vi "bottom stacking.vi"() -> (10 "Done":bool)   [LabVIEW 2014]
uses:
  Bottom Stacking.ctl
  <vilib>/Rock Robotics/WPI/RobotDrive/WPI_RobotDriveGetSetRefNum.vi
panel:
  out "Timer":dbl
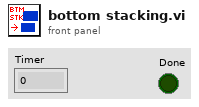
[diagram p1: front panel]
types:
  T1 = typedef "Bottom Stacking.ctl" = enum16{"Tote Raising", "Ejecting", "Un-Ejecting", "Tote Lowering", "Tote Release", "Backing Up"}
  T2 = typedef "WPI_RobotDriveDevRef.ctl" = cluster{"DevStatus":errorcluster, "Motors[]":T3[], "Square Inputs":bool, "Max Output":dbl}
  T3 = typedef "WPI_MotorControlDeviceRef.ctl" = cluster{"DeviceStatus":errorcluster, "Type":T4, "PWM":cluster{"Controller":T5, "PWM Channel":T6, "DeadBand":T7}, "CAN":cluster{"Device Number":u8, "Control Mode":T8, "Semaphore":T9, "Max Vout":dbl, "TalonSRX Control Mode":T10}, "Invert":bool, "TransformRef":T11, "InvTransformRef":T11}
  T4 = typedef "WPI_MotorControlType.ctl" = enum16{"PWM", "CAN", "CANTalonSRX"}
  T5 = typedef "FPGA_TypedefDigitalModule.ctl" = enum16{"Controller 1"}
  T6 = typedef "FPGA_DIOPWMChannel.ctl" = enum8{"PWM 0", "PWM 1", "PWM 2", "PWM 3", "PWM 4", "PWM 5", "PWM 6", "PWM 7", "PWM 8", "PWM 9", "PWM MXP 0", "PWM MXP 1", "PWM MXP 2", "PWM MXP 3", "PWM MXP 4", "PWM MXP 5", "PWM MXP 6", "PWM MXP 7", "PWM MXP 8", "PWM MXP 9", "Invalid"}
  T7 = typedef "WPI_PWMDeadband.ctl" = cluster{"Name":string, "maxPositivePwm":i32, "minPositivePwm":i32, "centerPwm":i32, "maxNegativePwm":i32, "minNegativePwm":i32, "angularRange":u16}
  T8 = typedef "WPI_CANJaguar_ControlMode.ctl" = enum8{"Percent VBus", "Current", "Speed", "Position", "Voltage"}
  T9 = typedef "Semaphore RefNum" = refnum<k1>
  T10 = typedef "WPI_CANTalonSRX_APIControlMode.ctl" = enum8{"Percent VBus", "Speed", "Position", "Slave", "Unchanged / Invalid"}
  T11 = typedef "WPI_PWMTransform_ConPane.ctl" = refnum<vi>
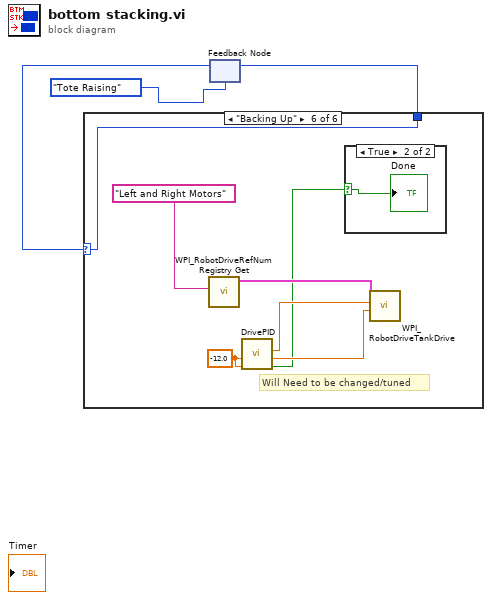
[diagram p0: block diagram]
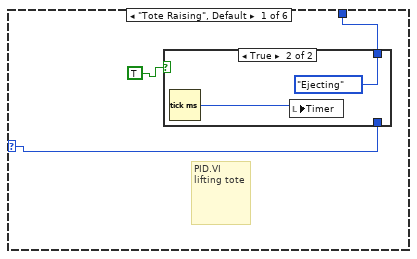
[diagram p2: hidden frame]
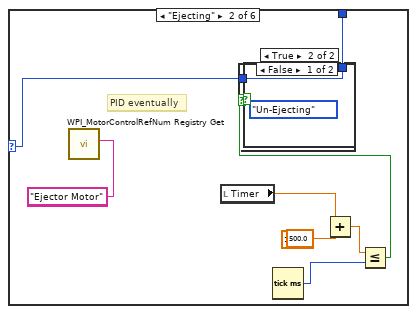
[diagram p4: hidden frame]
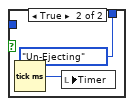
[diagram p5: hidden frame]
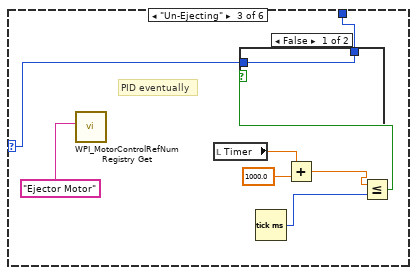
[diagram p7: hidden frame]
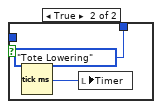
[diagram p8: hidden frame]
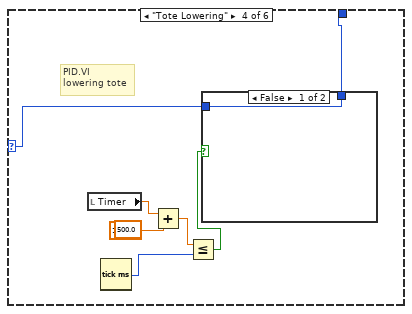
[diagram p9: hidden frame]
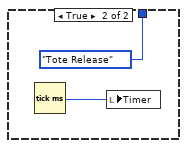
[diagram p10: hidden frame]
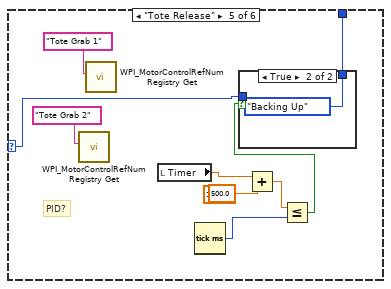
[diagram p11: hidden frame]
diagram:
  n1 = feedback #1(Bottom_Stacking."Tote Raising" ("Bottom Stacking")) -> (w2:T1)
  n2 = case shown="\"Backing Up\"" w2 {
    selector: w2 -> [w5 w10 w27 w37 w49 w58]
    tunnel: [w6 w11 w29 w43 w53 w58] -> w1
    frame "Tote Raising", Default {
      # "PID.VI\nlifting tote"
      n3 = case shown="True" TRUE {
        tunnel: [w7 Bottom_Stacking."Ejecting" ("Bottom Stacking")] -> w6
        tunnel: w5 -> [w7 _]
        frame False {
        }
        frame True {
          n4 = Tick Count (ms)() -> (millisecond timer value=w8:u32)
          n5 = local write "Timer"(w8) -> ()
        }
      }
    }
    frame "Ejecting" {
      (unwired) "Ejector Motor" ("refnum name")
      # "PID eventually"
      # "PID eventually"
      n6 = call <vilib>:"WPI_MotorControlRefNum Registry Get.vi"("refnum name"="Ejector Motor") -> ()  [unwired: 9 in, 2 out]
      n7 = local read "Timer"() -> (w21:dbl)
      n8 = local read "Timer"() -> (w12:dbl)
      n9 = Tick Count (ms)() -> (millisecond timer value=w18:u32)
      n10 = Tick Count (ms)() -> (millisecond timer value=w15:u32)
      n11 = Add(x=w21, y=500.0) -> (x+y=w19:dbl)
      n12 = Add(x=w12, y=1000.0) -> (x+y=w14:dbl)
      n13 = Less Or Equal?(x=w19, y=w18) -> (x <= y?=w17:bool)
      n14 = case shown="True" w17 {
        frame False {
        }
        frame True {
          (unwired) Bottom_Stacking."Un-Ejecting" ("Bottom Stacking")
        }
      }
      n15 = Less Or Equal?(x=w14, y=w15) -> (x <= y?=w16:bool)
      n16 = case shown="False" w16 {
        tunnel: [w23 Bottom_Stacking."Un-Ejecting" ("Bottom Stacking")] -> w11
        tunnel: w10 -> [w23 _]
        frame False {
        }
        frame True {
          n17 = Tick Count (ms)() -> (millisecond timer value=w25:u32)
          n18 = local write "Timer"(w25) -> ()
        }
      }
    }
    frame "Un-Ejecting" {
      # "PID eventually"
      n19 = call <vilib>:"WPI_MotorControlRefNum Registry Get.vi"("refnum name"="Ejector Motor") -> ()  [unwired: 9 in, 2 out]
      n20 = local read "Timer"() -> (w33:dbl)
      n21 = Tick Count (ms)() -> (millisecond timer value=w30:u32)
      n22 = Add(x=w33, y=1000.0) -> (x+y=w31:dbl)
      n23 = Less Or Equal?(x=w31, y=w30) -> (x <= y?=w28:bool)
      n24 = case shown="False" w28 {
        tunnel: [w34 Bottom_Stacking."Tote Lowering" ("Bottom Stacking")] -> w29
        tunnel: w27 -> [w34 _]
        frame False {
        }
        frame True {
          n25 = Tick Count (ms)() -> (millisecond timer value=w35:u32)
          n26 = local write "Timer"(w35) -> ()
        }
      }
    }
    frame "Tote Lowering" {
      (unwired) 500.0 ("y")
      # "PID.VI\nlowering tote"
      n27 = local read "Timer"() -> (w39:dbl)
      n28 = Tick Count (ms)() -> ()  [unwired: 1 out]
      n29 = Tick Count (ms)() -> (millisecond timer value=w40:u32)
      n30 = Add(x=w39, y=1000.0) -> (x+y=w41:dbl)
      n31 = Less Or Equal?(x=w41, y=w40) -> (x <= y?=w38:bool)
      n32 = case shown="False" w38 {
        tunnel: [w44 Bottom_Stacking."Tote Release" ("Bottom Stacking")] -> w43
        tunnel: w37 -> [w44 _]
        frame False {
        }
        frame True {
          n33 = Tick Count (ms)() -> (millisecond timer value=w45:u32)
          n34 = local write "Timer"(w45) -> ()
        }
      }
    }
    frame "Tote Release" {
      (unwired) 1000.0 ("y")
      # "PID?"
      n35 = call <vilib>:"WPI_MotorControlRefNum Registry Get.vi"("refnum name"="Tote Grab 2") -> ()  [unwired: 9 in, 2 out]
      n36 = call <vilib>:"WPI_MotorControlRefNum Registry Get.vi"("refnum name"="Tote Grab 1") -> ()  [unwired: 9 in, 2 out]
      n37 = local read "Timer"() -> (w48:dbl)
      n38 = Tick Count (ms)() -> (millisecond timer value=w52:u32)
      n39 = Tick Count (ms)() -> ()  [unwired: 1 out]
      n40 = Add(x=w48, y=500.0) -> (x+y=w51:dbl)
      n41 = Less Or Equal?(x=w51, y=w52) -> (x <= y?=w47:bool)
      n42 = case shown="True" w47 {
        tunnel: [w56 Bottom_Stacking."Backing Up" ("Bottom Stacking")] -> w53
        tunnel: w49 -> [w56 _]
        frame False {
        }
        frame True {
        }
      }
    }
    frame "Backing Up" {
      w60 = -12.0 ("SetpointLeft")
      # "Will Need to be changed/tuned"
      n43 = call <vilib>:"WPI_RobotDriveRefNum Registry Get.vi"("refnum name"="Left and Right Motors") -> ("RobotDriveDevRef"=w63:T2)  [unwired: 1 in, 9 out]
      n44 = call "DrivePID.vi"("SetpointLeft"=w60, "SetpointRight"=w60) -> ("Left Motor Output"=w62:dbl, "Right Motor Output"=w61:dbl, "Done"=w59:bool)  [unwired: 6 in]
      n45 = case shown="True" w59 {
        selector: w59 -> [_ w65]
        frame False {
        }
        frame True {
          "Done" <- w65
        }
      }
      n46 = call <vilib>:"WPI_RobotDriveTankDrive.vi"("Right axis value"=w61, "Left axis value"=w62, "RobotDriveDevRef"=w63) -> ()  [unwired: 6 in, 3 out]
    }
  }
  n47 = feedback-in #1(w1) -> ()
